vi "Remove Channel Group.vi"(8 "error in (no error)":errorcluster, 10 "name":string, 11 "FPGA Device in":refnum<class "FPGA Device.lvclass">) -> (0 "error out":errorcluster, 2 "found":bool, 3 "FPGA Device out":refnum<class "FPGA Device.lvclass">)   [LabVIEW 2016, in "FPGA RM Shared API.lvlib" / "FPGA Device.lvclass"]
uses:
  FPGA Device.lvclass
  FPGA Device.lvclass/FPGA Device.ctl
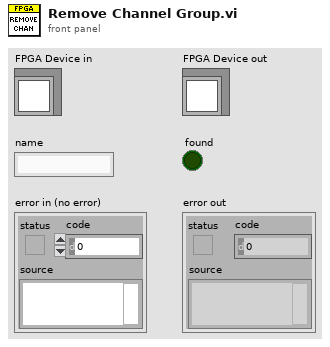
[diagram p1: front panel]
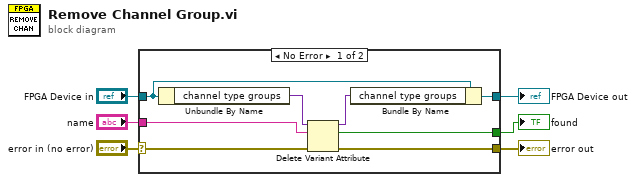
[diagram p0: block diagram]
diagram:
  n1 = case shown="No Error" "error in (no error)" {
    selector: "error in (no error)" -> [w8 w16]
    tunnel: [w7 w16] -> w5
    tunnel: [w13 w15] -> w3
    tunnel: "FPGA Device in" -> [w14 w15]
    tunnel: "name" -> [w11 _]
    tunnel: [w9 _] -> w1
    frame No Error {
      n2 = Unbundle By Name(w14) -> ("channel type groups"=w12:variant)
      n3 = Delete Variant Attribute(4:w8, 6:w11, 7:w12) -> (0:w7:errorcluster, 2:w9:bool, 3:w10:variant)
      n4 = Bundle By Name(cluster=w14, "channel type groups"=w10) -> (w13:refnum<class "FPGA Device.lvclass">)
    }
    frame Error {
    }
  }
  "error out" <- w5
  "FPGA Device out" <- w3
  "found" <- w1
